vi "Advanced Serial Write and Read.vi"(0 "VISA resource name":refnum<visa-resource-name>="COM1", 1 "baud rate":u32=9600, 4 "data bits":u16=8 min=5 max=8 step=1, 5 "parity":u16(ring) items=["None", "Odd", "Even", "Mark", "Space"], 7 "stop bits":u16(ring)=20 items=["1.0"=10, "1.5"=15, "2.0"=20], 15 "timeout (ms)":u32=10000, 17 "write INT":bool, 24 "termination char\n(0xA = '\\n' = LF)":u8=10 format="%.0x", 25 "Input\nbuffer size":u32=4096) -> ()   [LabVIEW 2017]
doc: "The Advanced Serial Read and Write example performs a Serial Port Read, a Serial Port Write, or a combination of these actions while setting some advanced serial features like buffer size, termination characters, and XON/XOFF flow control. The user selects the actions (read or write) on the front panel. If both are selected, the VI will write the data first, read the data and then close the VISA session that is opened to the port. \n\nThe parameters set for the serial port must match the parameters of the connected instrument or device. In this example, the bytes to read parameter specifies the number of bytes that the serial port reads. If there were more bytes at the port than the number specified in bytes to read, those bytes would not be read. Also, if you specify to read more bytes than the number of bytes actually read, you might receive a timeout error message.\n\nINSTRUCTIONS:\n1) Select the serial resource and configuration parameters (baud rate, data bits, parity, stop bits, flow control).\n2) Termination character can be enabled and set. Also, set the required input buffer size prior to running the example.\n3) Select the operations to be performed. \n4) Connect the serial port to your device. If no device is available, perform a loopback test by doing one of the following. Short pins 2 and 3 on a RS-232 cable or short pin 4 to pin 8 and pin 5 to pin 9 on a RS-485/422 cable. \n5) Run the VI to see the data read. (The \"read string\" will match the \"string to write\" if a loopback test was performed.)\n\nThis example exposes several advanced features that you may need for your application. Not all applications need all the features shown in this example. The input buffer size is likely an important setting that you want to control in your application. This example expands upon the flow control option for XON and XOFF, allowing the user to choose those control characters. The timeout parameter has been brought to the front panel so a user can specify the time period the VISA Read will wait for the number of bytes to read before timing out. Also, the user has several controls for the termination character, which is discussed later.\n\nNote that you can press the write and read buttons and change the bytes to read parameters on the fly, while the example is running. However, you must stop the example to change the other configuration parameters after the example has started running, and then run again.\n\nSet the I/O buffer size slightly higher the amount of data you expect to receive. This is very important for applications that don't use flow control, as you may lose characters if the receive buffer overflows.\n\nSetting the timeout period ensures that the operation returns with a timeout error if the operation cannot be performed in the specified time period. \n\nSome devices require a termination character in order to identify the end of command strings. Some devices send a termination character to signify the end of data to be read. \n\nThis example shows how you can end the Read operation once a termination character is detected in the buffer and/or append a termination character at the end of the Write data. To enable the Read to end on a termination character, use the VISA Configure Serial Port or use the VISA Properties Serial End Mode for Reads, Termination Character Enable, and Termination Character. To end the Write with a termination character, use the VISA Properties Serial End Mode for Writes, the Send End Enable, and Termination Character. In this example, the same termination character is used for both the Read and the Write. You can specify two different characters for your application, if desired.\n\nYour application may require specific characters for the XON/XOFF Flow Control. You can specify these characters with the VISA Properties Flow Control XOFF Character and Flow Control XON Character. Note that if the standard XON and XOFF characters are used, then decimal 17 and 19 are unavailable for data values. Remember that using flow control and setting an adequate buffer size allow you to prevent buffer overflows."
uses:
  Controls/Adresse.ctl
  TCxxxx.lvlib
panel:
  in  "Adresse":T1
  in  "update":bool
  out "Regler Rückgabewert\n[-32768 ... 32767]":i16
  in  "Parameter\n[0 ... 65535]":u16
  in  "Adresse":T1
  in  "Befehl \n[0 ... 65535]":u16
  in  "read INT":bool
  out "Regler Rückgabewert\n[0 ... 65535]":u16
  in  "Parameter\n[0 ... 65535]":u16
  in  "Adresse":T1
  in  "Befehl \n[0 ... 65535]":u16
  in  "read WORD":bool
  in  "Parameter\n[0 ... 65535]":u16
  in  "Adresse":T1
  in  "Befehl \n[0 ... 65535]":u16
  in  "write WORD":bool
  out "error out":errorcluster
  in  "Adresse":T1
  in  "Parameter \n[-32768 ... 0 ... 32767]":i16
  in  "Befehl \n[0 ... 65535]":u16
  in  "stop":bool
  in  "flow control":u16(ring) items=["None"=0, "XON/XOFF"=1, "RTS/CTS"=2, "DTR/DSR"=4]
  in  "End write with termination character?":bool
  # "For additional information select File >> VI Properties >> Documentation"
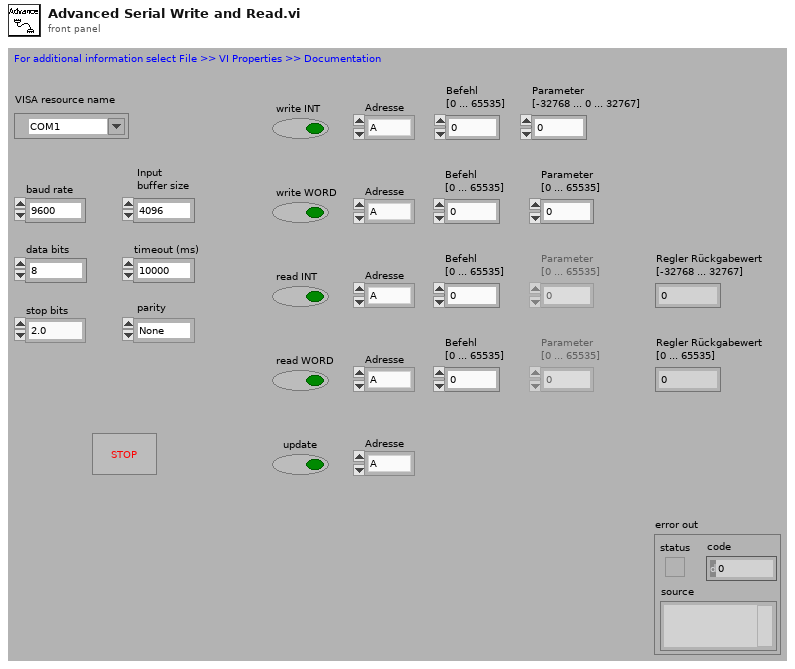
[diagram p1: front panel]
types:
  T1 = typedef "Adresse.ctl" = enum16{"A", "B", "C", "D", "E", "F", "G", "H", "I", "J", "K", "L", "M", "N", "O", "P", "Q", "R", "S", "T", "U", "V", "W", "X", "Y", "Z"}
  T2 = cluster{"Baud Rate":u32, "Parity":u16, "Data Bits":u16, "Stop Bits":u16, "Flow Control":u16}
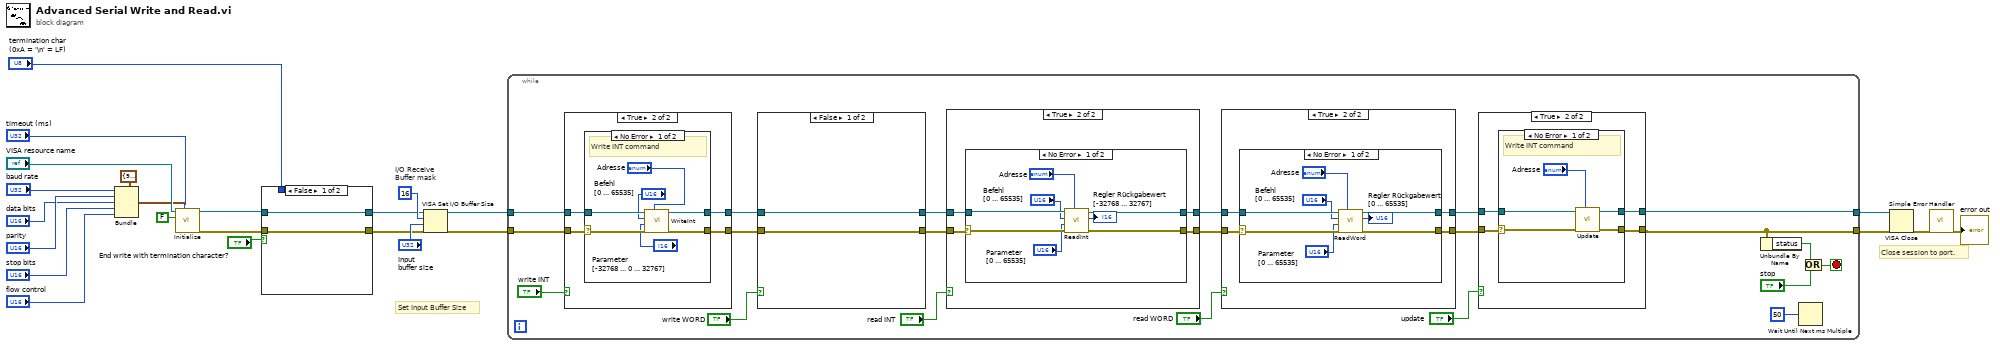
[diagram p0: block diagram]
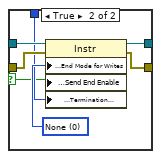
[diagram p2: hidden frame]
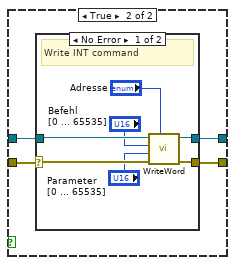
[diagram p7: hidden frame]
diagram:
  w23 = u16 16  # I/O Receive Buffer mask
  # "Set Input Buffer Size"
  # "Close session to port."
  n1 = Bundle(cluster=T2 {"Baud Rate"=9600, "Parity"=0, "Data Bits"=8, "Stop Bits"=20, "Flow Control"=0} ("Serial Configuration"), "Baud Rate"="baud rate", "Parity"="parity", "Data Bits"="data bits", "Stop Bits"="stop bits", "Flow Control"="flow control") -> (w8:T2)
  n2 = call "Initialize.vi"("Timeout [ms]"="timeout (ms)", "Serial Configuration"=w8, "ID Query (True)"=FALSE, "VISA resource name"="VISA resource name") -> ("error out"=w5:errorcluster, "VISA resource name out"=w6:refnum<visa-resource-name>)  [unwired: 6 in]
  n3 = case shown="False" "End write with termination character?" {
    selector: "End write with termination character?" -> [_ w27]
    tunnel: w6 -> [w25 w33]
    tunnel: w5 -> [w26 w32]
    tunnel: [w25 w31] -> w18
    tunnel: [w26 w30] -> w19
    tunnel: "termination char\n(0xA = '\\n' = LF)" -> [_ w28]
    frame False {
    }
    frame True {
      w29 = u16 0 items=["None", "LastBit", "TermChar", "Break"] ("Serial Settings:Serial End Mode for Writes")
      n4 = property class="Instr"(reference=w33, error in=w32, "Serial Settings:End Mode for Writes"=w29, "Message Based Settings:Send End Enable"=w27, "Message Based Settings:Termination Character"=w28) -> (reference out=w31:refnum<visa-resource-name>, error out=w30:errorcluster)
    }
  }
  n5 = VISA Set I/O Buffer Size(VISA resource name=w18, mask (16)=w23, size (4096)="Input\nbuffer size", error in (no error)=w19) -> (VISA resource name out=w2:refnum<visa-resource-name>, error out=w1:errorcluster)
  n6 = while {
    tunnel: w1 -> [w50]
    tunnel: w2 -> [w51]
    tunnel: [w35] -> w17
    tunnel: [w36] -> w16
    stop <- w49 stop-if-true
    n7 = case shown="True" "write INT" {
      tunnel: [w100 w104] -> w47
      tunnel: [w99 w103] -> w45
      tunnel: w51 -> [w100 w102]
      tunnel: w50 -> [w99 w101]
      frame False {
      }
      frame True {
        n8 = case shown="No Error" w101 {
          selector: w101 -> [w110 w113]
          tunnel: [w108 w112] -> w104
          tunnel: [w109 w113] -> w103
          tunnel: w102 -> [w111 w112]
          frame No Error {
            # "Write INT command"
            n9 = call "WriteInt.vi"("Adresse"="Adresse", "error in (no error)"=w110, "Parameter [-32768 ... 0 ... 32767]"="Parameter \n[-32768 ... 0 ... 32767]", "Befehl [0 ... 65535]"="Befehl \n[0 ... 65535]", "VISA resource name"=w111) -> ("error out"=w109:errorcluster, "VISA resource name out"=w108:refnum<visa-resource-name>)  [unwired: 4 in, 1 out]
          }
          frame Error {
          }
        }
      }
    }
    n10 = case shown="False" "write WORD" {
      tunnel: [w85 w89] -> w43
      tunnel: [w84 w88] -> w42
      tunnel: w47 -> [w85 w87]
      tunnel: w45 -> [w84 w86]
      frame False {
      }
      frame True {
        n11 = case shown="No Error" w86 {
          selector: w86 -> [w96 w98]
          tunnel: [w90 w97] -> w89
          tunnel: [w91 w98] -> w88
          tunnel: w87 -> [w95 w97]
          frame No Error {
            # "Write INT command"
            n12 = call "WriteWord.vi"("Adresse"="Adresse", "error in (no error)"=w96, "Parameter [0 ... 65535]"="Parameter\n[0 ... 65535]", "Befehl [0 ... 65535]"="Befehl \n[0 ... 65535]", "VISA resource name"=w95) -> ("error out"=w91:errorcluster, "VISA resource name out"=w90:refnum<visa-resource-name>)  [unwired: 4 in, 1 out]
          }
          frame Error {
          }
        }
      }
    }
    n13 = case shown="True" "read INT" {
      tunnel: w42 -> [w68 w71]
      tunnel: w43 -> [w69 w70]
      tunnel: [w68 w73] -> w40
      tunnel: [w69 w72] -> w41
      frame False {
      }
      frame True {
        n14 = case "Read bytes from port." shown="No Error" w71 {
          selector: w71 -> [w80 w82]
          tunnel: [w79 w82] -> w73
          tunnel: [w78 w83] -> w72
          tunnel: w70 -> [w81 w83]
          frame No Error {
            n15 = call "ReadInt.vi"("Adresse"="Adresse", "error in (no error)"=w80, "Parameter [0 ... 65535]"="Parameter\n[0 ... 65535]", "Befehl [0 ... 65535]"="Befehl \n[0 ... 65535]", "VISA resource name"=w81) -> ("error out"=w79:errorcluster, "Regler Rückgabewert [-32768 ... 32767]"=→"Regler Rückgabewert\n[-32768 ... 32767]":i16, "VISA resource name out"=w78:refnum<visa-resource-name>)  [unwired: 3 in, 1 out]
          }
          frame Error {
            # "Error occurred \nreading Bytes at \nSerial Port"
          }
        }
      }
    }
    n16 = case shown="True" "read WORD" {
      tunnel: w40 -> [w114 w118]
      tunnel: w41 -> [w115 w117]
      tunnel: [w114 w116] -> w37
      tunnel: [w115 w119] -> w38
      frame False {
      }
      frame True {
        n17 = case "Read bytes from port." shown="No Error" w118 {
          selector: w118 -> [w126 w128]
          tunnel: [w124 w128] -> w116
          tunnel: [w125 w129] -> w119
          tunnel: w117 -> [w127 w129]
          frame No Error {
            n18 = call "ReadWord.vi"("Adresse"="Adresse", "error in (no error)"=w126, "Parameter [0 ... 65535]"="Parameter\n[0 ... 65535]", "Befehl [0 ... 65535]"="Befehl \n[0 ... 65535]", "VISA resource name"=w127) -> ("error out"=w124:errorcluster, "Regler Rückgabewert [0 ... 65535]"=→"Regler Rückgabewert\n[0 ... 65535]":u16, "VISA resource name out"=w125:refnum<visa-resource-name>)  [unwired: 3 in, 1 out]
          }
          frame Error {
            # "Error occurred \nreading Bytes at \nSerial Port"
          }
        }
      }
    }
    n19 = case shown="True" "update" {
      tunnel: [w56 w60] -> w35
      tunnel: [w55 w59] -> w36
      tunnel: w38 -> [w56 w58]
      tunnel: w37 -> [w55 w57]
      frame False {
      }
      frame True {
        n20 = case shown="No Error" w57 {
          selector: w57 -> [w64 w67]
          tunnel: [w63 w66] -> w60
          tunnel: [w62 w67] -> w59
          tunnel: w58 -> [w65 w66]
          frame No Error {
            # "Write INT command"
            n21 = call "Update.vi"("Adresse"="Adresse", "error in (no error)"=w64, "VISA resource name"=w65) -> ("error out"=w62:errorcluster, "VISA resource name out"=w63:refnum<visa-resource-name>)  [unwired: 7 in]
          }
          frame Error {
          }
        }
      }
    }
    n22 = Unbundle By Name(w36) -> ("status"=w53:bool)
    n23 = Wait Until Next ms Multiple(millisecond multiple=u32 50) -> ()  [unwired: 1 out]
    n24 = Or(x=w53, y="stop") -> (x .or. y?=w49:bool)
  }
  n25 = VISA Close(VISA resource name=w17, error in (no error)=w16) -> (error out=w24:errorcluster)
  n26 = call <vilib>:"Simple Error Handler.vi"("error in (no error)"=w24) -> ("error out"=→"error out":errorcluster)  [unwired: 1 in, 7 out]
